vi "Close Instrument.vi"(1 "Instrument Prop":T1={"Public"={"Column Name"=[], "Trace Color"=[]}, "Private"={"Path"=path "", "VI Refnum"=refnum, "Name"="", "# of Values"=0, "Scale Factors"=[], "Display"=[], "Offset"=[1.0]}} {"Private"."Offset" format="%^_3e"; "Private"."Scale Factors" format="%^_3e"}) -> (0 "Instrument Prop 2":T1={"Public"={"Column Name"=[], "Trace Color"=[]}, "Private"={"Path"=path "", "VI Refnum"=refnum, "Name"="", "# of Values"=0, "Scale Factors"=[], "Display"=[], "Offset"=[1.0]}} {"Private"."Offset" format="%^_3e"; "Private"."Scale Factors" format="%^_3e"})   [LabVIEW 2019]
uses:
  Sub Controls/Instrument Properties.ctl
  Sub Controls/Public.ctl
  Sub Controls/Private.ctl
  Sub Controls/Instrument Ref.ctl
  Sub Controls/SystemCheckBox-resize.ctl
  Sub Controls/Instrument Actions.ctl
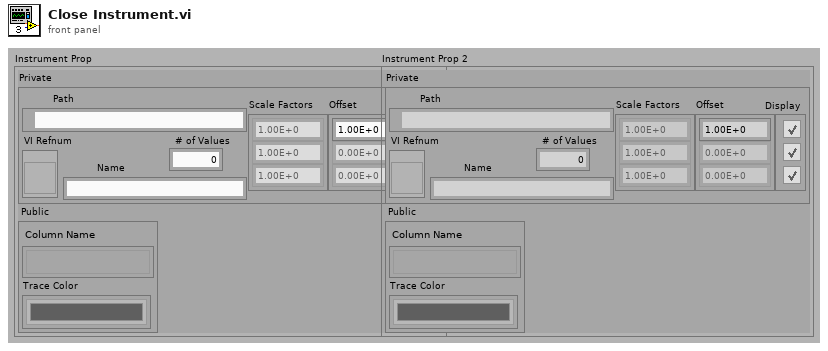
[diagram p1: front panel]
types:
  T1 = typedef "Instrument Properties.ctl" = cluster{"Public":T2, "Private":T3}
  T2 = typedef "Public.ctl" = cluster{"Column Name":string[], "Trace Color":u32[]}
  T3 = typedef "Private.ctl" = cluster{"Path":path, "VI Refnum":T4, "Name":string, "# of Values":i32, "Scale Factors":dbl[], "Display":T5[], "Offset":dbl[]}
  T4 = typedef "Instrument Ref.ctl" = refnum<vi>
  T5 = typedef "SystemCheckBox-resize.ctl" = bool
  T6 = typedef "Instrument Actions.ctl" = enum16{"Scan", "Identify", "New", "Configure", "Initialize", "Test", "Read", "Close"}
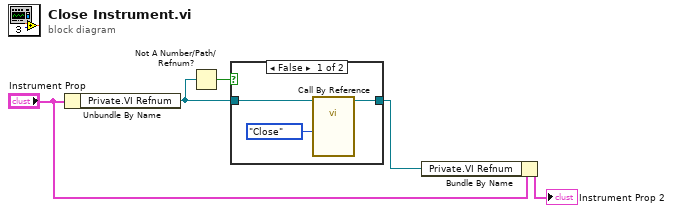
[diagram p0: block diagram]
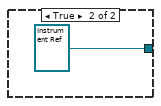
[diagram p2: hidden frame]
diagram:
  n1 = Unbundle By Name("Instrument Prop") -> ("Private.VI Refnum"=w5:T4)
  n2 = Not A Number/Path/Refnum?(number/path/refnum=w5) -> (NaN/Path/Refnum?=w4:bool)
  n3 = case shown="False" w4 {
    tunnel: w5 -> [w7 _]
    tunnel: [w6 T4 refnum ("VI Refnum")] -> w1
    frame False {
      n4 = call-by-ref "?"(reference=w7, "Action"=Instrument_Actions."Close") -> (reference out=w6:T4)  [unwired: 6 in, 3 out]
    }
    frame True {
    }
  }
  n5 = Bundle By Name(cluster="Instrument Prop", "Private.VI Refnum"=w1) -> (→"Instrument Prop 2":T1)
